vi "Initialize board layout.vi"(1 "Board implementation":refnum<class "Board.lvclass">) -> (0 "Initialized board":refnum<class "Board.lvclass">)   [LabVIEW 2015, in "Chesslib.lvlib" / "Position.lvclass"]
uses:
  Position.lvclass
  Board/Board.lvclass
  typedef/Square.ctl
  typedef/File.ctl
  typedef/Rank.ctl
  typedef/Piece.ctl
  typedef/Color.ctl
  typedef/Piece type.ctl
  Chesslib.lvlib
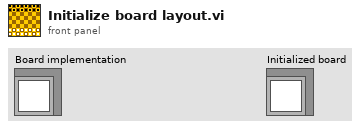
[diagram p1: front panel]
types:
  T1 = typedef "Chesslib.lvlib/Square.ctl" = cluster{"File":T2, "Rank":T3}
  T2 = typedef "Chesslib.lvlib/File.ctl" = enum16{"a", "b", "c", "d", "e", "f", "g", "h"}
  T3 = typedef "Chesslib.lvlib/Rank.ctl" = enum16{"1", "2", "3", "4", "5", "6", "7", "8"}
  T4 = typedef "Chesslib.lvlib/Piece.ctl" = cluster{"Color":T5, "Type":T6}
  T5 = typedef "Chesslib.lvlib/Color.ctl" = enum16{"White", "Black"}
  T6 = typedef "Chesslib.lvlib/Piece type.ctl" = enum16{"Pawn", "Bishop", "Knight", "Rook", "Queen", "King"}
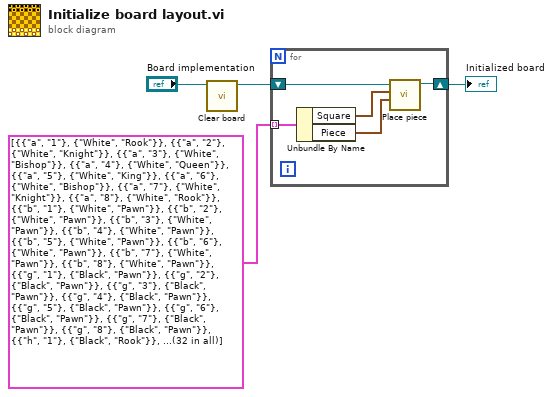
[diagram p0: block diagram]
diagram:
  n1 = call-dynamic "Clear board.vi"("Board in"="Board implementation") -> ("Board out"=w2:refnum<class "Board.lvclass">)  [unwired: 9 in, 1 out]
  n2 = for {
    tunnel: cluster{"Square":T1, "Piece":T4}[] [{"Square"={"File"=enum."a", "Rank"=enum."1"}, "Piece"={"Color"=enum."White", "Type"=enum."Rook"}}, {"Square"={"File"=enum."a", "Rank"=enum."2"}, "Piece"={"Color"=enum."White", "Type"=enum."Knight"}}, {"Square"={"File"=enum."a", "Rank"=enum."3"}, "Piece"={"Color"=enum."White", "Type"=enum."Bishop"}}, {"Square"={"File"=enum."a", "Rank"=enum."4"}, "Piece"={"Color"=enum."White", "Type"=enum."Queen"}}, {"Square"={"File"=enum."a", "Rank"=enum."5"}, "Piece"={"Color"=enum."White", "Type"=enum."King"}}, {"Square"={"File"=enum."a", "Rank"=enum."6"}, "Piece"={"Color"=enum."White", "Type"=enum."Bishop"}}, {"Square"={"File"=enum."a", "Rank"=enum."7"}, "Piece"={"Color"=enum."White", "Type"=enum."Knight"}}, {"Square"={"File"=enum."a", "Rank"=enum."8"}, "Piece"={"Color"=enum."White", "Type"=enum."Rook"}}, {"Square"={"File"=enum."b", "Rank"=enum."1"}, "Piece"={"Color"=enum."White", "Type"=enum."Pawn"}}, {"Square"={"File"=enum."b", "Rank"=enum."2"}, "Piece"={"Color"=enum."White", "Type"=enum."Pawn"}}, {"Square"={"File"=enum."b", "Rank"=enum."3"}, "Piece"={"Color"=enum."White", "Type"=enum."Pawn"}}, {"Square"={"File"=enum."b", "Rank"=enum."4"}, "Piece"={"Color"=enum."White", "Type"=enum."Pawn"}}, {"Square"={"File"=enum."b", "Rank"=enum."5"}, "Piece"={"Color"=enum."White", "Type"=enum."Pawn"}}, {"Square"={"File"=enum."b", "Rank"=enum."6"}, "Piece"={"Color"=enum."White", "Type"=enum."Pawn"}}, {"Square"={"File"=enum."b", "Rank"=enum."7"}, "Piece"={"Color"=enum."White", "Type"=enum."Pawn"}}, {"Square"={"File"=enum."b", "Rank"=enum."8"}, "Piece"={"Color"=enum."White", "Type"=enum."Pawn"}}, {"Square"={"File"=enum."g", "Rank"=enum."1"}, "Piece"={"Color"=enum."Black", "Type"=enum."Pawn"}}, {"Square"={"File"=enum."g", "Rank"=enum."2"}, "Piece"={"Color"=enum."Black", "Type"=enum."Pawn"}}, {"Square"={"File"=enum."g", "Rank"=enum."3"}, "Piece"={"Color"=enum."Black", "Type"=enum."Pawn"}}, {"Square"={"File"=enum."g", "Rank"=enum."4"}, "Piece"={"Color"=enum."Black", "Type"=enum."Pawn"}}, {"Square"={"File"=enum."g", "Rank"=enum."5"}, "Piece"={"Color"=enum."Black", "Type"=enum."Pawn"}}, {"Square"={"File"=enum."g", "Rank"=enum."6"}, "Piece"={"Color"=enum."Black", "Type"=enum."Pawn"}}, {"Square"={"File"=enum."g", "Rank"=enum."7"}, "Piece"={"Color"=enum."Black", "Type"=enum."Pawn"}}, {"Square"={"File"=enum."g", "Rank"=enum."8"}, "Piece"={"Color"=enum."Black", "Type"=enum."Pawn"}}, {"Square"={"File"=enum."h", "Rank"=enum."1"}, "Piece"={"Color"=enum."Black", "Type"=enum."Rook"}}, {"Square"={"File"=enum."h", "Rank"=enum."2"}, "Piece"={"Color"=enum."Black", "Type"=enum."Knight"}}, {"Square"={"File"=enum."h", "Rank"=enum."3"}, "Piece"={"Color"=enum."Black", "Type"=enum."Bishop"}}, {"Square"={"File"=enum."h", "Rank"=enum."4"}, "Piece"={"Color"=enum."Black", "Type"=enum."Queen"}}, {"Square"={"File"=enum."h", "Rank"=enum."5"}, "Piece"={"Color"=enum."Black", "Type"=enum."King"}}, {"Square"={"File"=enum."h", "Rank"=enum."6"}, "Piece"={"Color"=enum."Black", "Type"=enum."Bishop"}}, {"Square"={"File"=enum."h", "Rank"=enum."7"}, "Piece"={"Color"=enum."Black", "Type"=enum."Knight"}}, {"Square"={"File"=enum."h", "Rank"=enum."8"}, "Piece"={"Color"=enum."Black", "Type"=enum."Rook"}}] ("Board layout") -> [w7] mode=indexing
    shift-right: [w8] -> w1
    shift-left: w2 -> [w9]
    n3 = Unbundle By Name(w7) -> ("Square"=w6:T1, "Piece"=w5:T4)
    n4 = call-dynamic "Place piece.vi"("Piece"=w5, "Square"=w6, "Board in"=w9) -> ("Board out"=w8:refnum<class "Board.lvclass">)  [unwired: 5 in, 3 out]
  }
  "Initialized board" <- w1
